vi "Tenney TON timer.vi"(8 "error in (no error)":errorcluster, 11 "Time Target (s)":dbl=1.0) -> (0 "error out":errorcluster, 2 "Elapsed Time (s)":dbl, 3 "Time has Elapsed":bool)   [LabVIEW 2023]
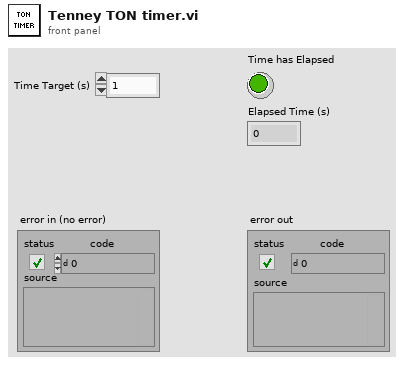
[diagram p1: front panel]
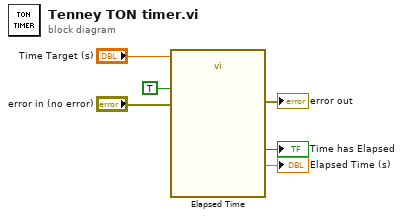
[diagram p0: block diagram]
diagram:
  n1 = call "Elapsed Time"("Time Target (s)"="Time Target (s)", "Auto Reset"=TRUE, "error in (no error)"="error in (no error)") -> ("Elapsed Time (s)"=→"Elapsed Time (s)":dbl, "Time has Elapsed"=→"Time has Elapsed":bool, "error out"=→"error out":errorcluster)  [unwired: 9 in, 5 out]
